vi "Recursion Solution.vi"() -> ()   [LabVIEW 2018]
uses:
  ctl/Coin data--cluster.ctl
panel:
  out "Max Quantities":i32[](array[numeric])
  out "Solutions (Quantity)":i32[][](array[numeric])
  out "No. solutions":i32
  out "Values (£)":i32[](array[numeric])
  out "Time taken (s)":dbl
  # "Beer money - Recursion Solution"
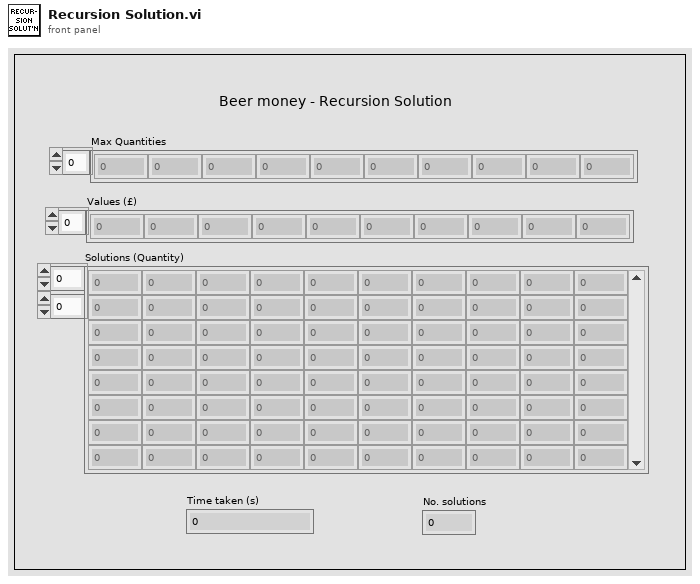
[diagram p1: front panel]
types:
  T1 = typedef "Coin data--cluster.ctl" = cluster{"Coin/note":i32, "Quantity":i32}
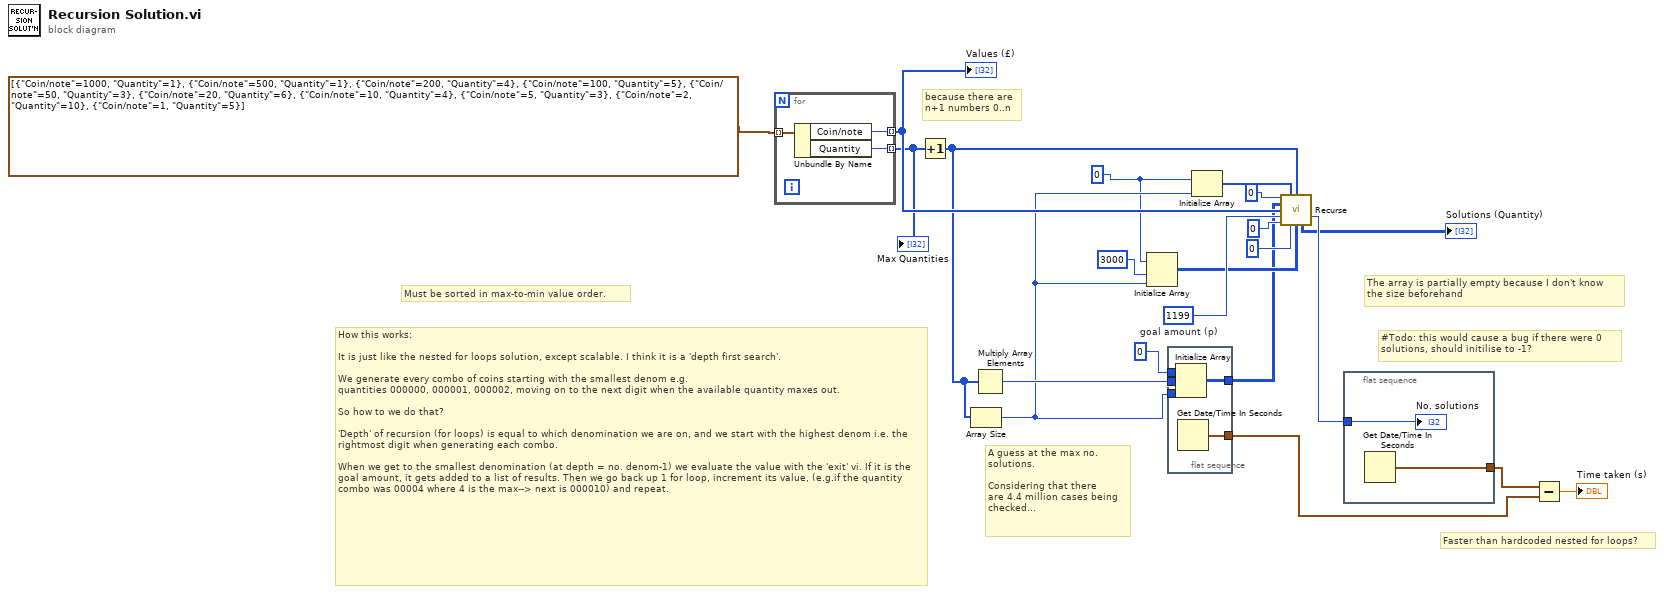
[diagram p0: block diagram]
diagram:
  w9 = 1199  # goal amount (p)
  w10 = 0
  # "Faster than hardcoded nested for loops?"
  # "How this works:\n\nIt is just like the nested for loops solution, except scalable. I think it is a 'depth first search'.\n\nWe generate every combo of coins starting with the smallest denom e.g.\nquantities 000000, 000001, 000002, moving on to the next digit when the available quantity maxes out.\n\nSo how to we do that?\n\n'Depth' of recursion (for loops) is equal to which denomination we are on, and we start with the highest denom i.e. the rightmost digit when generating each combo.\n\nWhen we get to the smallest denomination (at depth = no. denom-1) we evaluate the value with the 'exit' vi. If it is the goal amount, it gets added to a list of results. Then we go back up 1 for loop, increment its value, (e.g.if the quantity combo was 00004 where 4 is the max--> next is 000010) and repeat."
  # "A guess at the max no.\nsolutions.\n\nConsidering that there \nare 4.4 million cases being \nchecked..."
  # "#Todo: this would cause a bug if there were 0\nsolutions, should initilise to -1?"
  # "Must be sorted in max-to-min value order."
  # "The array is partially empty because I don't know\nthe size beforehand"
  # "because there are \nn+1 numbers 0..n"
  n1 = for {
    tunnel: T1[] [{"Coin/note"=1000, "Quantity"=1}, {"Coin/note"=500, "Quantity"=1}, {"Coin/note"=200, "Quantity"=4}, {"Coin/note"=100, "Quantity"=5}, {"Coin/note"=50, "Quantity"=3}, {"Coin/note"=20, "Quantity"=6}, {"Coin/note"=10, "Quantity"=4}, {"Coin/note"=5, "Quantity"=3}, {"Coin/note"=2, "Quantity"=10}, {"Coin/note"=1, "Quantity"=5}] -> [w24] mode=indexing
    tunnel: [w23] -> w17 mode=indexing
    tunnel: [w22] -> w1 mode=indexing
    n2 = Unbundle By Name(w24) -> ("Coin/note"=w23:i32, "Quantity"=w22:i32)
  }
  "Values (£)" <- w17
  "Max Quantities" <- w1
  n3 = Increment(x=w1) -> (x+1=w14:i32[])
  n4 = Array Size(array=w14) -> (size(s)=w15:i32)
  n5 = Multiply Array Elements(1:w14) -> (0:w21:i32)
  n6 = Initialize Array(w10, 3000 ("dimension size"), w15) -> (w7:i32[][])
  n7 = flat-sequence {
    tunnel: w21 -> [w29]
    tunnel: [w28] -> w20
    tunnel: w15 -> [w27]
    tunnel: 0 ("dimension size") -> [w26]
    tunnel: [w25] -> w4
    frame #0 {
      n8 = Initialize Array(w26, w29, w27) -> (w25:i32[][])
      n9 = Get Date/Time In Seconds() -> (seconds since 1Jan1904=w28:timestamp)
    }
  }
  n10 = Initialize Array(w10, w15) -> (w13:i32[])
  n11 = call "Recurse.vi"("Combo index in"=0 ("combo index in"), "Iterations array in"=w13, "Quantities"=w14, "Combos in"=w4, "Values"=w17, "Goal amount"=w9, "Depth"=0, "Result index in"=0 ("result index in"), "Results in"=w7) -> ("Result index out"=w16:i32, "Results out"=→"Solutions (Quantity)":i32[][])  [unwired: 2 in, 3 out]
  n12 = flat-sequence {
    tunnel: [w31] -> w19
    tunnel: w16 -> [w30]
    frame #0 {
      n13 = Get Date/Time In Seconds() -> (seconds since 1Jan1904=w31:timestamp)
      "No. solutions" <- w30
    }
  }
  n14 = Subtract(x=w19, y=w20) -> (x-y=→"Time taken (s)":dbl)
